vi "Actor Core.vi"(8 "error in":errorcluster, 11 "Test Executive Builder View In":refnum<class "Test Executive Builder View.lvclass">) -> (0 "error out":errorcluster, 3 "Actor out":refnum<class "Actor.lvclass">)   [LabVIEW 2017, in "Test Executive Builder View.lvclass"]
doc: "(<B>Filename</B>: Actor Framework.lvlib:Actor.lvclass:Actor Core.vi)\n\nReceives messages to the actor, reacts to them, and initiates any error handling that may shut the actor down.\n\nDescendant classes may override this VI to append parallel tasks for the actor to complete while it handles messages. Overrides use the Call Parent Method node.\n\n<License>\nCopyright © 2017 Composed Systems, LLC | All rights reserved\nwww.composed.io\n\nAuthor: Ethan Stern <ethan.stern@composed.io>\n\nThis software is provided \"AS IS\" WITHOUT WARRANTIES, either express or implied, AND IS FOR EDUCATIONAL PURPOSES ONLY.\n</License>"
uses:
  Test Executive Builder View.lvclass
  C:/Program Files/National Instruments/LabVIEW 2017/vi.lib/gpm_packages/@cs/mva-viewable/Source/ActorEvents/IEventAggregator/IEventAggregator.lvclass
  C:/Program Files/National Instruments/LabVIEW 2017/vi.lib/ActorFramework/Actor/Actor.lvclass
  <vilib>/ActorFramework/Actor/Actor.lvclass
  Test Executive Builer Event Filter/Test Executive Builder Event Filter.lvclass
  C:/Program Files/National Instruments/LabVIEW 2017/vi.lib/gpm_packages/@cs/mva-viewable/Source/ActorEvents/IEventFilter/IEventFilter.lvclass
  <vilib>/event_ctls.llb/lveventtype.ctl
  Test Executive Builder View.lvclass/Test Executive Builder View.ctl
  <vilib>/ActorFramework/Actor/Actor.lvclass/Actor.ctl
  <vilib>/ActorFramework/Message Enqueuer/Message Enqueuer.lvclass/Message Enqueuer.ctl
  Test Executive Builer Event Filter/Test Executive Builder Event Filter.lvclass/Test Executive Builder Event Filter.ctl
  <vilib>/ActorFramework/Message Enqueuer/Init from Existing Queue.vi
  <vilib>/ActorFramework/Message Enqueuer/Message Enqueuer.lvclass
  <vilib>/gpm_packages/@cs/mva-viewable/Source/IViewable/IViewable/IViewable.lvclass
  <vilib>/gpm_packages/@cs/mva-viewable/Source/ActorEvents/IEventAggregator/IEventAggregator.lvclass
  <vilib>/gpm_packages/@cs/mva-viewable/Source/ActorEvents/IEventFilter/IEventFilter.lvclass
  Test Executive Builder View Messages/Populate Menu Msg/Populate Menu Msg.lvclass
  Test Executive Builder View Messages/Handle Mouse Down Msg/Handle Mouse Down Msg.lvclass
  Test Executive Builder View Messages/Handle Drag Starting Msg/Handle Drag Starting Msg.lvclass
  Test Executive Builder View Messages/Handle Drop Msg/Handle Drop Msg.lvclass
  Test Executive Builder View Messages/Handle Drag Over Msg/Handle Drag Over Msg.lvclass
panel:
  out "Alpha Mask":bool
  in  "Test Executive":string(tree)
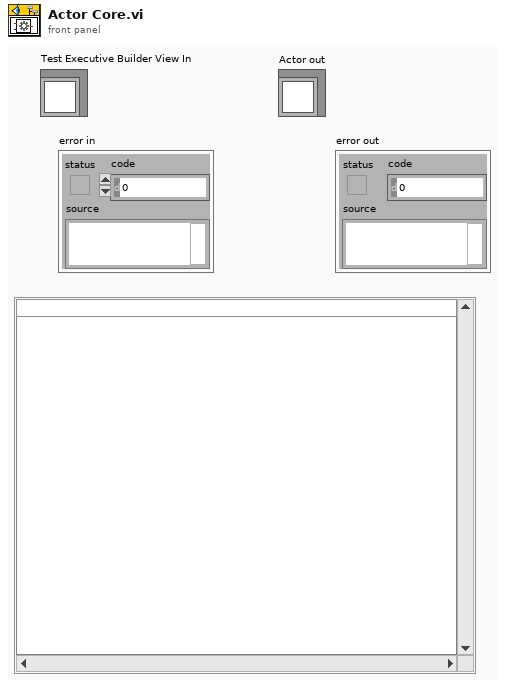
[diagram p1: front panel]
types:
  T1 = typedef "lveventtype.ctl" = enum32{"Null", "Timeout", "Annotation Menu Selection", "Annotation Menu Selection?", "App Instance Close", "App Instance Close?", "Autoscale Range Change", "Bookmark Info Change", "Cell Edit", "Cell Edit?", "Cursor Grab", "Cursor Grab?", "Cursor Menu Selection", "Cursor Menu Selection?", "Cursor Move", "Cursor Release", "Data Change", "Direction Change", "Display State Change", "Drag Ended", "Drag Enter", "Drag Leave", "Drag Over", "Drag Source Update", "Drag Starting", "Drag Starting?", "Drop", "Exec State Change", "Key Down", "Key Down?", "Key Repeat", "Key Repeat?", "Key Up", "Listbox Double Click", "Menu Activation?", "Menu Selection (App)", "Menu Selection? (App)", "Menu Selection (User)", "Mouse Down", "Mouse Down?", "Mouse Enter", "Mouse Leave", "Mouse Move", "Mouse Up", "Mouse Wheel", "NI Security User Change (App)", "Pane Size", "Panel Close", "Panel Close?", "Panel Resize", "Plot Attribute Change", "Scale Range Change", "Shortcut Menu Activation?", "Shortcut Menu Selection (App)", "Shortcut Menu Selection? (App)", "Shortcut Menu Selection (User)", "Tree Double Click", "Tree Drag", "Tree Drag?", "Tree Drop", "Tree Drop?", "Tree Item Close", "Tree Item Close?", "Tree Item Open", "Tree Item Open?", "User Event", "Value Change"}
  T2 = typedef "ActorEvents.lvlib/IEventFilter.lvclass/EventFilter Reference.ctl" = refnum<data-value>
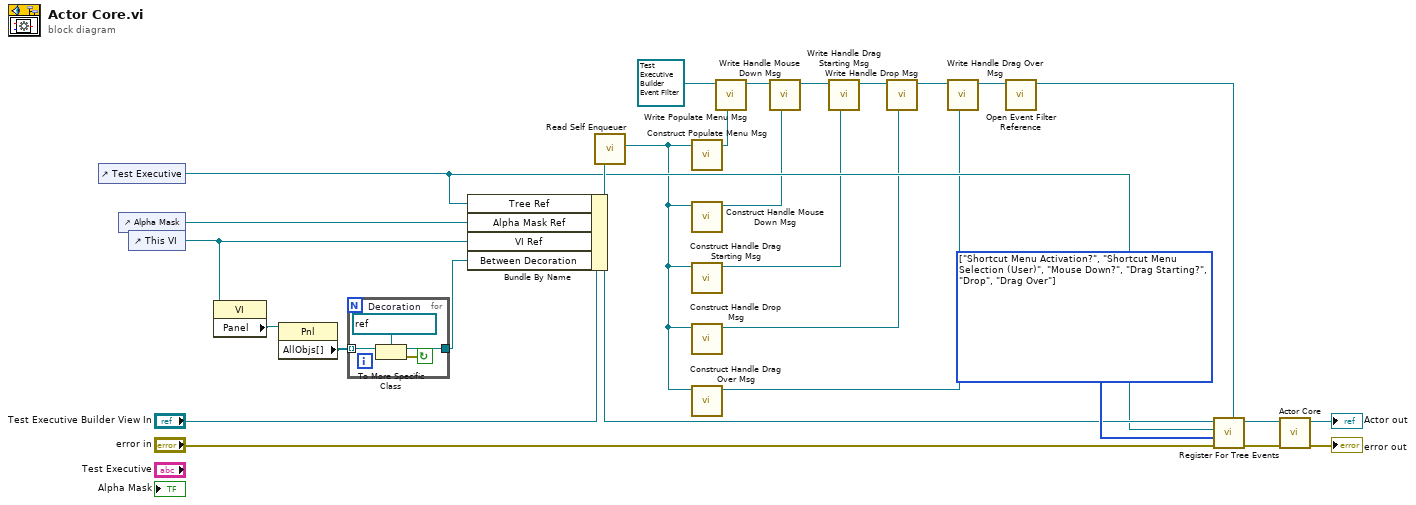
[diagram p0: block diagram]
diagram:
  w20 = T1[] [enum."Shortcut Menu Activation?", enum."Shortcut Menu Selection (User)", enum."Mouse Down?", enum."Drag Starting?", enum."Drop", enum."Drag Over"] items=["Null", "Timeout", "Annotation Menu Selection", "Annotation Menu Selection?", "App Instance Close", "App Instance Close?", "Autoscale Range Change", "Bookmark Info Change", "Cell Edit", "Cell Edit?", "Cursor Grab", "Cursor Grab?", "Cursor Menu Selection", "Cursor Menu Selection?", "Cursor Move", "Cursor Release", "Data Change", "Direction Change", "Display State Change", "Drag Ended", "Drag Enter", "Drag Leave", "Drag Over", "Drag Source Update", "Drag Starting", "Drag Starting?", "Drop", "Exec State Change", "Key Down", "Key Down?", "Key Repeat", "Key Repeat?", "Key Up", "Listbox Double Click", "Menu Activation?", "Menu Selection (App)", "Menu Selection? (App)", "Menu Selection (User)", "Mouse Down", "Mouse Down?", "Mouse Enter", "Mouse Leave", "Mouse Move", "Mouse Up", "Mouse Wheel", "NI Security User Change (App)", "Pane Size", "Panel Close", "Panel Close?", "Panel Resize", "Plot Attribute Change", "Scale Range Change", "Shortcut Menu Activation?", "Shortcut Menu Selection (App)", "Shortcut Menu Selection? (App)", "Shortcut Menu Selection (User)", "Tree Double Click", "Tree Drag", "Tree Drag?", "Tree Drop", "Tree Drop?", "Tree Item Close", "Tree Item Close?", "Tree Item Open", "Tree Item Open?", "User Event", "Value Change"] ("Registration Types")
  n1 = control-ref of="Test Executive"() -> (w8:refnum<vi>)
  n2 = control-ref of="Alpha Mask"() -> (w9:refnum<vi>)
  n3 = control-ref of="This VI"() -> (w11:refnum<vi>)
  n4 = property class="VI"(reference=w11) -> ("Panel"=w13:refnum<vi>)  [unwired: 1 in, 2 out]
  n5 = property class="Pnl"(reference=w13) -> ("AllObjs[]"=w12:refnum<vi>[])  [unwired: 1 in, 2 out]
  n6 = for {
    tunnel: w12 -> [w31] mode=indexing
    tunnel: [w29] -> w7
    stop <- w30 continue-if-true
    w28 = refnum<vi> refnum  # Decoration
    n7 = To More Specific Class(target class=w28, reference=w31) -> (specific class reference=w29:refnum<vi>, error out=w30:errorcluster)  [unwired: 1 in]
  }
  n8 = Bundle By Name(cluster="Test Executive Builder View In", "Tree Ref"=w8, "Alpha Mask Ref"=w9, "VI Ref"=w11, "Between Decoration"=w7) -> (w10:refnum<class "Test Executive Builder View.lvclass">)
  n9 = call <vilib>:"Read Self Enqueuer.vi"("Actor"=w10) -> ("Self Enqueuer"=w1:refnum<class "Message Enqueuer.lvclass">)  [unwired: 10 in]
  n10 = call "Construct Populate Menu Msg.vi"("Return Enqueuer"=w1) -> ("Populate Menu Msg out"=w6:refnum<class "Populate Menu Msg.lvclass">)  [unwired: 10 in]
  n11 = call "Construct Handle Mouse Down Msg.vi"("Return Enqueuer"=w1) -> ("Handle Mouse Down Msg out"=w5:refnum<class "Handle Mouse Down Msg.lvclass">)  [unwired: 10 in]
  n12 = call "Construct Handle Drag Starting Msg.vi"("Return Enqueuer"=w1) -> ("Handle Drag Starting Msg out"=w4:refnum<class "Handle Drag Starting Msg.lvclass">)  [unwired: 10 in]
  n13 = call "Construct Handle Drop Msg.vi"("Return Enqueuer"=w1) -> ("Handle Drop Msg out"=w3:refnum<class "Handle Drop Msg.lvclass">)  [unwired: 10 in]
  n14 = call "Construct Handle Drag Over Msg.vi"("Return Enqueuer"=w1) -> ("Handle Drag Over Msg out"=w2:refnum<class "Handle Drag Over Msg.lvclass">)  [unwired: 10 in]
  n15 = call "Write Populate Menu Msg.vi"("Populate Menu Msg"=w6, "Test Executive Builder Event Filter in"=refnum<class "Test Executive Builder Event Filter.lvclass"> refnum ("Test Executive Builder View.lvlib:Test Executive Builder Event Filter.lvclass")) -> ("Test Executive Builder Event Filter out"=w18:refnum<class "Test Executive Builder Event Filter.lvclass">)  [unwired: 9 in]
  n16 = call "Write Handle Mouse Down Msg.vi"("Handle Mouse Down Msg"=w5, "Test Executive Builder Event Filter in"=w18) -> ("Test Executive Builder Event Filter out"=w17:refnum<class "Test Executive Builder Event Filter.lvclass">)  [unwired: 9 in]
  n17 = call "Write Handle Drag Starting Msg.vi"("Handle Drag Starting Msg"=w4, "Test Executive Builder Event Filter in"=w17) -> ("Test Executive Builder Event Filter out"=w16:refnum<class "Test Executive Builder Event Filter.lvclass">)  [unwired: 9 in]
  n18 = call "Write Handle Drop Msg.vi"("Handle Drop Msg"=w3, "Test Executive Builder Event Filter in"=w16) -> ("Test Executive Builder Event Filter out"=w15:refnum<class "Test Executive Builder Event Filter.lvclass">)  [unwired: 9 in]
  n19 = call "Write Handle Drag Over Msg.vi"("Handle Drag Over Msg"=w2, "Test Executive Builder Event Filter in"=w15) -> ("Test Executive Builder Event Filter out"=w14:refnum<class "Test Executive Builder Event Filter.lvclass">)  [unwired: 9 in]
  n20 = call <vilib>:"Open Event Filter Reference.vi"("IEventFilter in"=w14) -> ("IEventFilter Reference"=w21:T2)  [unwired: 9 in, 1 out]
  n21 = call <vilib>:"Register For Tree Events.vi"("EventFilter Reference"=w21, "error in (no error)"="error in", "Registration Types"=w20, "Tree Refnum"=w8, "IEventAggregator In"=w10) -> ("error out"=w23:errorcluster, "IEventAggregator Out"=w22:refnum<class "Test Executive Builder View.lvclass">)  [unwired: 5 in]
  n22 = call-parent "Actor Core.vi"("error in"=w23, "IViewable In"=w22) -> ("error out"=→"error out":errorcluster, "Actor out"=→"Actor out":refnum<class "Actor.lvclass">)  [unwired: 8 in]
